vi "Test Report.vi"(8 "error in (no error)":errorcluster, 10 "Test Log":i32(ring) items=["Baseboard", "SubModule1", "SubModule2"], 11 "Instrument Handle In":i32(ring)) -> (0 "error out":errorcluster, 2 "Report":string, 3 "Instrument Handle Out":i32(ring))   [LabVIEW 8.6, in "ZTScopeM.lvlib"]
doc: "Returns the next self test report entry for the specified log."
uses:
  ZTScopeM.lvlib
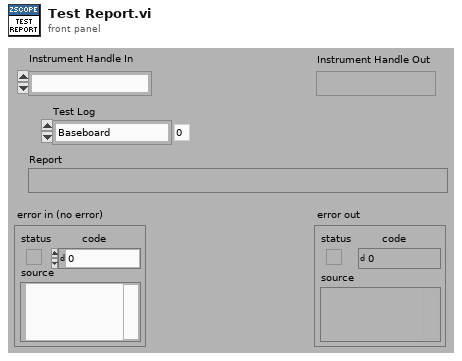
[diagram p1: front panel]
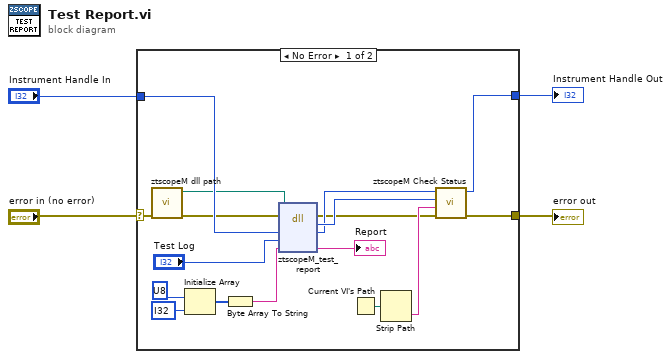
[diagram p0: block diagram]
diagram:
  n1 = case shown="No Error" "error in (no error)" {
    selector: "error in (no error)" -> [w8 w23]
    tunnel: [w18 w23] -> w3
    tunnel: "Instrument Handle In" -> [w20 w22]
    tunnel: [w19 w22] -> w1
    frame #0 {
      n2 = call "ztscopeM dll path.vi"("error in (no error)"=w8) -> ("error out"=w6:errorcluster, "<instrument>.dll path"=w7:path)  [unwired: 9 in]
      n3 = Initialize Array(u8 ?, i32 ? ("dimension size")) -> (w11:u8[])
      n4 = Byte Array To String(unsigned byte array=w11) -> (string=w9:string)
      n5 = dll-call lib="C:/Program Files (x86)/National Instruments/LabVIEW 2013/instr.lib/ztscopem/ztscopeM.dll" fn="ztscopeM_test_report"(path in=w7, error in=w6, "Instrument Handle"=w20, "Test Log"="Test Log", "Report"=w9) -> (error out=w5:errorcluster, "Status"=w16:i32, "Instrument Handle"=w15:i32, "Report"=→"Report":string)  [unwired: 2 in, 1 out]
      n6 = Current VI's Path() -> (path=w21:path)
      n7 = Strip Path(path=w21) -> (name=w17:string)  [unwired: 1 out]
      n8 = call "ztscopeM Check Status.vi"("error in"=w5, "name of VI"=w17, "status (return code)"=w16, "instrument handle in"=w15) -> ("error out"=w18:errorcluster, "instrument handle out"=w19:i32)  [unwired: 2 in]
    }
    frame #1 {
    }
  }
  "error out" <- w3
  "Instrument Handle Out" <- w1
